vi "Set Cell Border.vi"(4 "Column":i32=-1, 6 "Row":i32=-1, 9 "Width":i32(ring)=2 items=["None"=0, "Thin"=2], 10 "Edge":i32(ring)=9 items=["Top"=8, "Bottom"=9, "Left"=7, "Right"=10], 11 "Excel Sheet in":refnum<class "Excel Sheet.lvclass">) -> (3 "Excel Sheet out":refnum<class "Excel Sheet.lvclass">)   [LabVIEW 2016, in "Excel Sheet.lvclass"]
uses:
  Excel Sheet.lvclass
panel:
  out "error out":errorcluster
  in  "error in (no error)":errorcluster
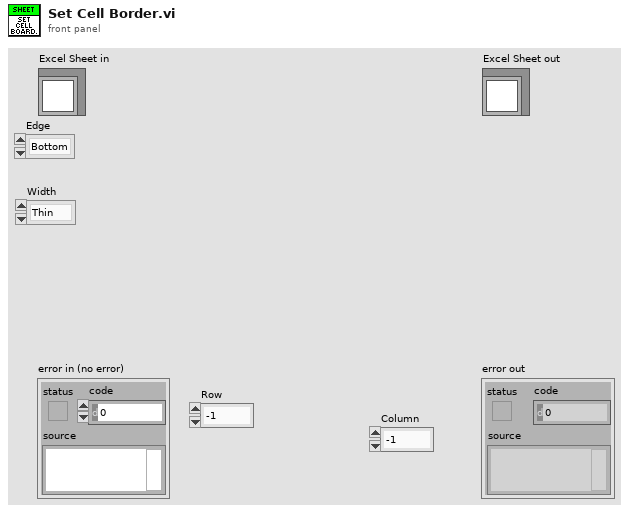
[diagram p1: front panel]
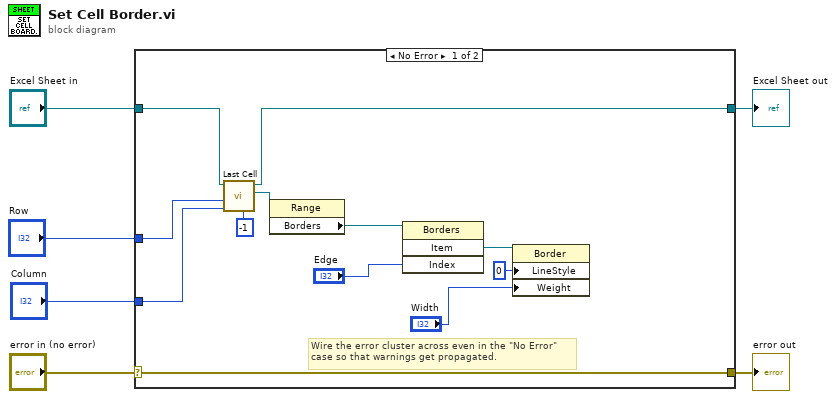
[diagram p0: block diagram]
diagram:
  n1 = case shown="No Error" "error in (no error)" {
    selector: "error in (no error)" -> [w18 w20]
    tunnel: [w18 w20] -> w5
    tunnel: [w16 w19] -> w3
    tunnel: "Excel Sheet in" -> [w17 w19]
    tunnel: "Column" -> [w13 _]
    tunnel: "Row" -> [w12 _]
    frame No Error {
      # "Wire the error cluster across even in the \"No Error\"\ncase so that warnings get propagated."
      n2 = call "Last Cell.vi"("Col Offset"=-1, "Column"=w13, "Row"=w12, "Excel Sheet in"=w17) -> ("Cell"=w14:refnum<k7>, "Excel Sheet out"=w16:refnum<class "Excel Sheet.lvclass">)  [unwired: 4 in, 2 out]
      n3 = property class="Range"(reference=w14) -> ("Borders"=w11:refnum<k7>)  [unwired: 1 in, 2 out]
      n4 = invoke class="Borders" method="Item"(reference=w11, "Index"="Edge") -> ("Item"=w10:refnum<k7>)  [unwired: 2 in, 3 out]
      n5 = property class="Border"(reference=w10, "LineStyle"=0, "Weight"="Width") -> ()  [unwired: 1 in, 2 out]
    }
    frame Error {
    }
  }
  "error out" <- w5
  "Excel Sheet out" <- w3
